vi "Configure Relays.vi"(4 "Alarm Type (0:Low)":u16(ring) items=["Low", "High", "Both"], 6 "Mode (0:Off)":enum16{"Off", "On", "Alarms"}(ring), 8 "error in (no error)":errorcluster, 9 "Input (0)":i32 min=0 max=7 step=1, 10 "Relay (0)":i32=1 min=0 max=7 step=1, 11 "LS218 in":refnum<class "LS218.lvclass">) -> (0 "error out":errorcluster, 3 "LS218 out":refnum<class "LS218.lvclass">)   [LabVIEW 2013, in "LS218.lvlib" / "LS218.lvclass"]
doc: "This VI configures relay paramters. Relays may be configured manually or set to activate on an input alarm condition. Only the model 218S includes the relays."
uses:
  LS218.lvclass
  LS218.lvclass/LS218.ctl
  <instrlib>/Lake Shore Cryotronics 218/Lake Shore Cryotronics 218.lvlib
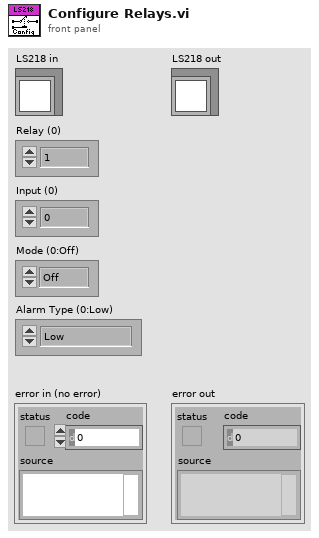
[diagram p1: front panel]
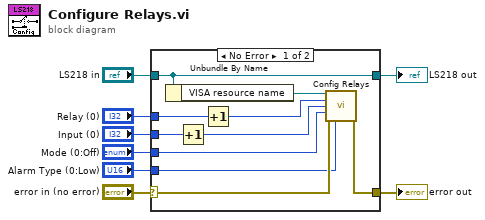
[diagram p0: block diagram]
diagram:
  n1 = case shown="No Error" "error in (no error)" {
    selector: "error in (no error)" -> [w11 w20]
    tunnel: [w10 w20] -> w7
    tunnel: [w18 w19] -> w5
    tunnel: "LS218 in" -> [w18 w19]
    tunnel: "Input (0)" -> [w17 _]
    tunnel: "Relay (0)" -> [w14 _]
    tunnel: "Mode (0:Off)" -> [w12 _]
    tunnel: "Alarm Type (0:Low)" -> [w9 _]
    frame No Error {
      n2 = Unbundle By Name(w18) -> ("VISA resource name"=w16:refnum<visa-resource-name>)
      n3 = Increment(x=w17) -> (x+1=w15:i32)
      n4 = Increment(x=w14) -> (x+1=w13:i32)
      n5 = call <instrlib>:"Config Relays.vi"("VISA resource name"=w16, "Relay (1)"=w13, "Input (1)"=w15, "Mode (0:Off)"=w12, "error in (no error)"=w11, "Alarm Type (0:Off)"=w9) -> ("error out"=w10:errorcluster)  [unwired: 8 in, 1 out]
    }
    frame Error {
    }
  }
  "error out" <- w7
  "LS218 out" <- w5
